vi "Initialize.vi"(7 "ProjectItem":refnum<class "ProjectItem.lvclass">, 8 "error in (no error)":errorcluster, 10 "New Name":string="NewName", 11 "Pattern":string="[Rename]") -> (0 "error out":errorcluster, 3 "ProjectItem out":refnum<class "ProjectItem.lvclass">)   [LabVIEW 2019, in "ProjectItem.lvclass"]
uses:
  ProjectItem.lvclass
  ProjectItem.lvclass/ProjectItem.ctl
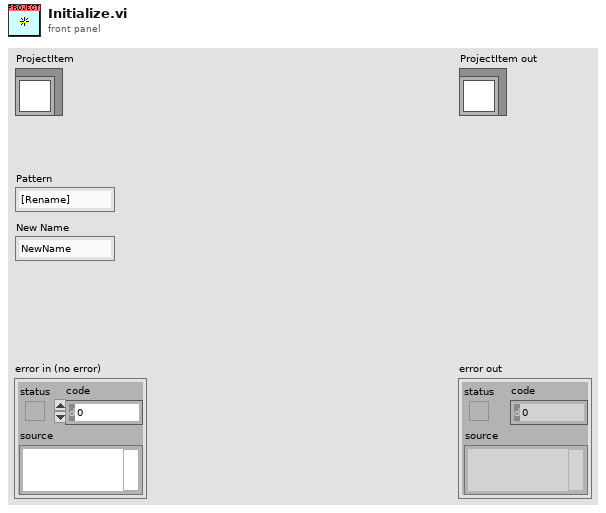
[diagram p1: front panel]
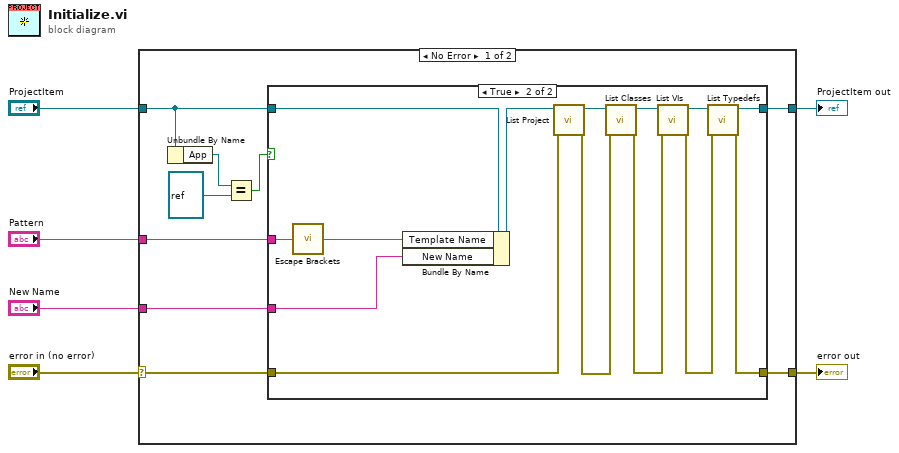
[diagram p0: block diagram]
diagram:
  n1 = case shown="No Error" "error in (no error)" {
    selector: "error in (no error)" -> [w15 w33]
    tunnel: [w13 w33] -> w5
    tunnel: [w14 w32] -> w3
    tunnel: "ProjectItem" -> [w10 w32]
    tunnel: "Pattern" -> [w12 _]
    tunnel: "New Name" -> [w11 _]
    frame No Error {
      n2 = Unbundle By Name(w10) -> ("App"=w9:refnum<vi>)
      n3 = Equal?(x=w9, y=refnum<vi> refnum ("App")) -> (x = y?=w8:bool)
      n4 = case shown="True" w8 {
        tunnel: w15 -> [w16 w25]
        tunnel: [w17 w20] -> w14
        tunnel: [w16 w18] -> w13
        tunnel: w12 -> [_ w31]
        tunnel: w11 -> [_ w22]
        tunnel: w10 -> [w17 w24]
        frame False {
        }
        frame True {
          n5 = call "Escape Brackets.vi"("Pattern"=w31) -> ("result string"=w26:string)
          n6 = Bundle By Name(cluster=w24, "Template Name"=w26, "New Name"=w22) -> (w23:refnum<class "ProjectItem.lvclass">)
          n7 = call "List Project.vi"("error in (no error)"=w25, "Rename in"=w23) -> ("error out"=w27:errorcluster, "Rename out"=w30:refnum<class "ProjectItem.lvclass">)  [unwired: 8 in]
          n8 = call "List Classes.vi"("error in (no error)"=w27, "Rename in"=w30) -> ("error out"=w28:errorcluster, "Rename out"=w29:refnum<class "ProjectItem.lvclass">)  [unwired: 8 in]
          n9 = call "List VIs.vi"("error in (no error)"=w28, "Rename in"=w29) -> ("error out"=w19:errorcluster, "Rename out"=w21:refnum<class "ProjectItem.lvclass">)  [unwired: 8 in]
          n10 = call "List Typedefs.vi"("error in (no error)"=w19, "Rename in"=w21) -> ("error out"=w18:errorcluster, "Rename out"=w20:refnum<class "ProjectItem.lvclass">)  [unwired: 8 in]
        }
      }
    }
    frame Error {
    }
  }
  "error out" <- w5
  "ProjectItem out" <- w3
